vi "WPI_Power Get 5Volt Rail Voltage and Current.vi"(11 "error in":errorcluster) -> (6 "5 volt rail voltage (V)":dbl, 8 "5 volt rail current (A)":dbl, 15 "error out":errorcluster)   [LabVIEW 2017]
doc: "Returns the voltage and current of the 5 volt user rail on the roboRIO in the robot program. On the roboRIO the 5 volt rail is connected to:\npin V of DIO channels (internal jumper set to 5V)\npin V of ANALOG IN channels\npin 5V of SPI\npin 1 of MXP"
uses:
  <vilib>/Utility/error.llb/Error Cluster From Error Code.vi
  <vilib>/rvi/errors/niLvFpgaAdjustHostInterfaceError.vi
  <vilib>/rvi/interface/nirviReadWriteControl/nirviReadWriteControl.xnode
  <vilib>/Rock Robotics/SystemInterfaces/System/FPGA_SystemFRC FPGA Ref.ctl
  NiFpgaLv.dll
  <vilib>/rvi/interface/Simulation/niFpgaSimulationCallBeginRW.vi
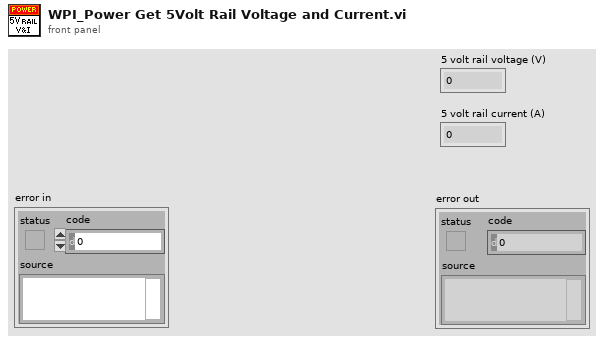
[diagram p1: front panel]
types:
  T1 = typedef "FPGA_SystemFRC FPGA Ref.ctl" = refnum<k20>
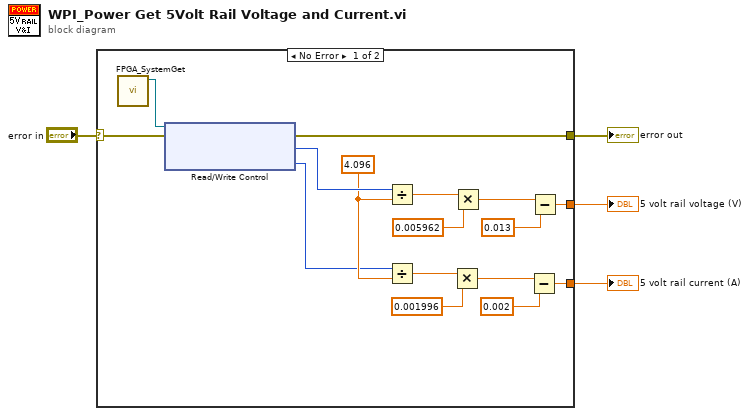
[diagram p0: block diagram]
diagram:
  n1 = case shown="No Error" "error in" {
    selector: "error in" -> [w6 w21]
    tunnel: [w7 w21] -> w3
    tunnel: [w17 _] -> w2
    tunnel: [w13 _] -> w1
    frame No Error {
      w8 = 4.096 ("battery voltage out")
      n2 = call <vilib>:"FPGA_SystemGet.vi"() -> ("FRC FPGA Ref"=w11:T1)  [unwired: 2 in, 9 out]
      n3 = xnode "Read/Write Control"("FPGA VI Reference In"=w11, "error in"=w6) -> ("error out"=w7:errorcluster, "Power.UserVoltage5V"=w12:u16, "Power.UserCurrent5V"=w5:u16)  [unwired: 1 out]
      n4 = Divide(x=w12, y=w8) -> (x/y=w10:dbl)
      n5 = Divide(x=w5, y=w8) -> (x/y=w9:dbl)
      n6 = Multiply(x=w9, y=0.001996 ("battery voltage out")) -> (x*y=w15:dbl)
      n7 = Multiply(x=w10, y=0.005962 ("battery voltage out")) -> (x*y=w19:dbl)
      n8 = Subtract(x=w15, y=0.002 ("battery voltage out")) -> (x-y=w13:dbl)
      n9 = Subtract(x=w19, y=0.013 ("battery voltage out")) -> (x-y=w17:dbl)
    }
    frame Error {
    }
  }
  "error out" <- w3
  "5 volt rail voltage (V)" <- w2
  "5 volt rail current (A)" <- w1
